vi "Mass Flow Control 8 Ch Subvi.vi"(0 "LINX In":T1, 8 "VISA resource name":refnum<visa-resource-name>="COM5", 10 "Servo Channel":u8=11, 11 "MFC 8 set point":dbl, 13 "MFC 7 set point":dbl, 14 "MFC 1  set point":dbl, 15 "MFC 2 set point":dbl, 16 "MFC 3 set point":dbl, 17 "MFC 4 set point":dbl, 18 "MFC 5 set point":dbl, 19 "MFC 6 set point":dbl) -> (12 "LINX Out":T1)   [LabVIEW 2013]
uses:
  647 Multi Gas Controller.llb/647 Open/Close Valve .vi
  <vilib>/MakerHub/LINX/Public/Sensors/Motion/Servo/Servo.lvlib
  <vilib>/Instr/_visa.llb/VISA Configure Serial Port (Instr).vi
  <vilib>/MakerHub/LINX/Public/Sensors/Motion/Servo/Servo Set Pulse Width One Channel.vi
  <vilib>/MakerHub/LINX/Private/Type Defs/Platform.ctl
  <vilib>/MakerHub/LINX/LMH-LINX.lvlib
  <vilib>/MakerHub/LINX/Private/Type Defs/Interface.ctl
  <vilib>/MakerHub/LINX/Private/Device/Type Defs/TCP Config.ctl
  <vilib>/MakerHub/LINX/Private/Device/Device.lvlib
  <vilib>/MakerHub/LINX/Private/Device/Type Defs/Channels.ctl
  <vilib>/MakerHub/LINX/Private/Device/Type Defs/LINX Device Config.ctl
  <vilib>/MakerHub/LINX/Private/Type Defs/LINX Ref.ctl
panel:
  in  "Off":dbl=1900.0
  in  "On":dbl=860.0
  out "GCF 8":dbl=1.0
  out "GCF 7":dbl=1.0
  out "GCF 6":dbl=1.0
  out "MFC 8 Size":dbl=1.0
  out "MFC 7 Size":dbl=1.0
  out "MFC 6 Size":dbl=1.0
  out "MFC 8 Status":bool
  out "MFC 7 Status":bool
  out "MFC 6 Status":bool
  out "GCF 5":dbl=0.94
  out "GCF 4":dbl=1.01
  out "GCF 3":dbl=1.22
  out "GCF 2":dbl=0.9
  out "GCF 1":dbl=0.95
  out "MFC 5 Size":dbl=100.0
  out "MFC 4 Size":dbl=50.0
  out "MFC 3 Size":dbl=50.0
  out "MFC 2 Size":dbl=100.0
  out "MFC 1 Size":dbl=50.0
  out "MFC 5 Status":bool
  out "MFC 4 Status":bool
  out "MFC 1 Status":bool
  out "MFC 2 Status":bool
  out "MFC 3 Status":bool
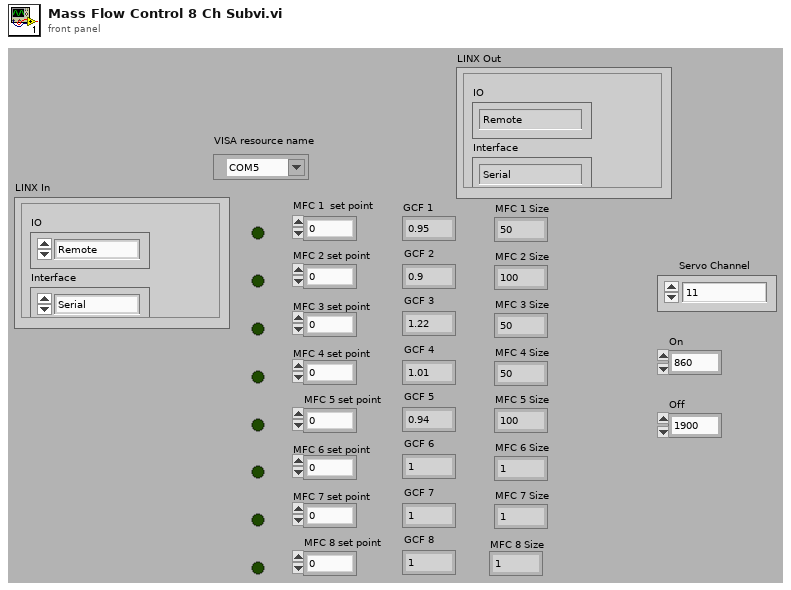
[diagram p1: front panel]
types:
  T1 = typedef "LMH-LINX.lvlib/LINX Ref.ctl" = cluster{"IO":T2, "Interface":T3, "LINX Device Config":T4}
  T2 = typedef "LMH-LINX.lvlib/Platform.ctl" = enum16{"Remote", "Local"}
  T3 = typedef "LMH-LINX.lvlib/Interface.ctl" = enum16{"Serial", "TCP"}
  T4 = typedef "LMH-LINX.lvlib/Device.lvlib/LINX Device Config.ctl" = cluster{"Interface":T3, "COM Port":refnum<visa-resource-name>, "TCP Configuration":T5, "Device Family":u8, "Device ID":u8, "Device Name":string, "TCP Ref":refnum<k5>, "Channels":T6}
  T5 = typedef "LMH-LINX.lvlib/Device.lvlib/TCP Config.ctl" = cluster{"IP Address":string, "Port":u16}
  T6 = typedef "LMH-LINX.lvlib/Channels.ctl" = cluster{"DI":u8[], "DO":u8[], "AI":u8[], "AO":u8[], "PWM":u8[], "QE":u8[], "UART":u8[], "I2C 2":u8[], "SPI":u8[], "CAN":u8[], "Servo":u8[], "AI Ref (V)":dbl, "AI Resolution (Bits)":u8, "AO Ref (V)":dbl, "AO Resolution (Bits)":u8}
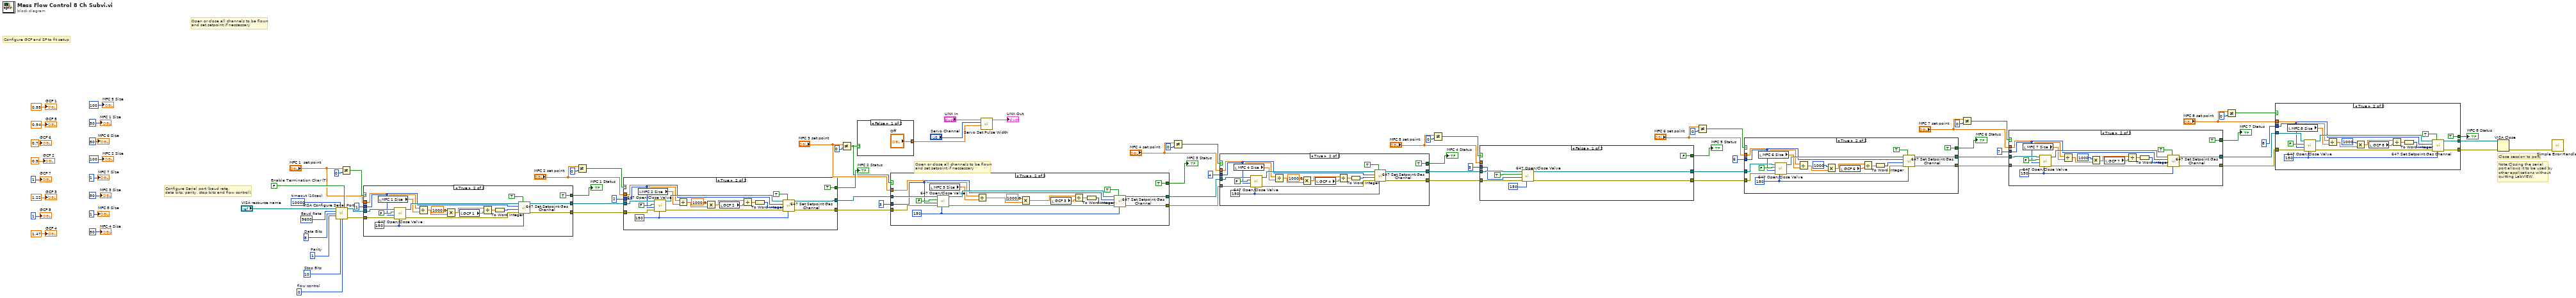
[diagram p0: block diagram]
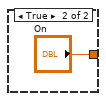
[diagram p2: hidden frame]
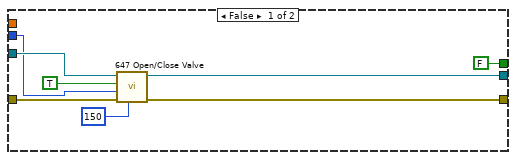
[diagram p3: hidden frame]
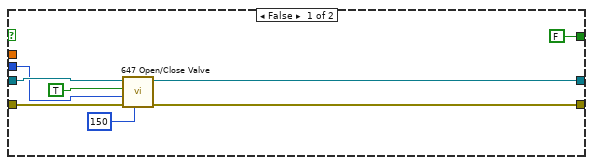
[diagram p4: hidden frame]
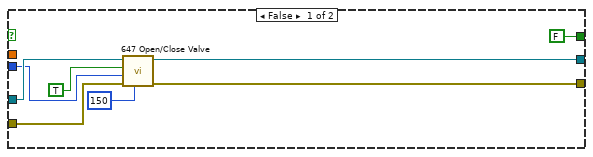
[diagram p5: hidden frame]
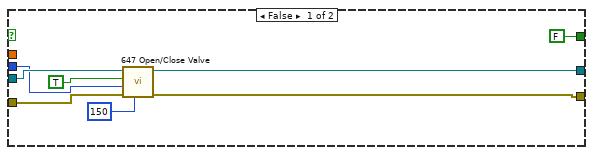
[diagram p6: hidden frame]
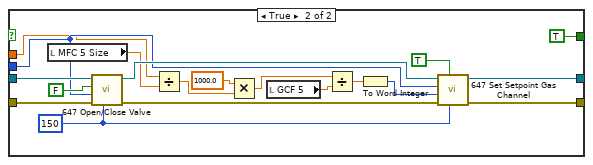
[diagram p7: hidden frame]
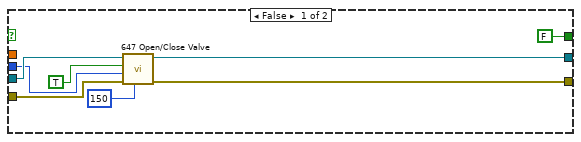
[diagram p8: hidden frame]
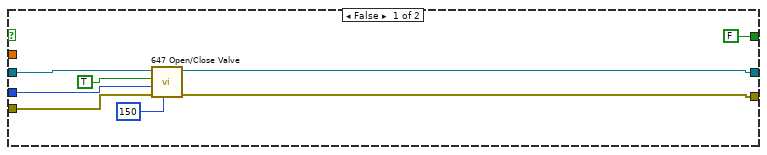
[diagram p9: hidden frame]
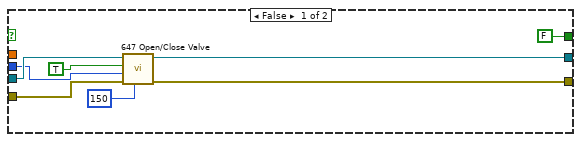
[diagram p10: hidden frame]
diagram:
  w80 = 0  # flow control
  w81 = 10  # Stop Bits
  w82 = 1  # Parity
  w83 = 8  # Data Bits
  w84 = 9600  # Baud Rate
  w85 = FALSE  # Enable Termination Char (T)
  w86 = u32 10000  # timeout (10sec)
  # "Open or close all channels to be flown\nand set setpoint if neccessary"
  # "Open or close all channels to be flown\nand set setpoint if neccessary"
  # "Configure GCF and SF to fit setup"
  # "Note:Closing the serial port allows it to be used by other applications without\nquitting LabVIEW."
  # "Close session to port."
  # "Configure Serial port (baud rate,\ndata bits, parity, stop bits and flow control)."
  n1 = call-poly "VISA Configure Serial Port"("VISA resource name"="VISA resource name", "timeout (10sec)"=w86, "Enable Termination\nChar (T)"=w85, "baud rate (9600)"=w84, "data bits (8)"=w83, "parity (0:none)"=w82, "stop bits (10: 1 bit)"=w81, "flow control (0:none)"=w80) -> ("VISA resource name out"=w79:refnum<visa-resource-name>, "error out"=w78:errorcluster)  [unwired: 6 in]
  n2 = Not Equal?(x="MFC 1  set point", y=0) -> (x != y?=w26:bool)
  n3 = case shown="True" w26 {
    tunnel: w78 -> [w91 w114]
    tunnel: [w92 w109] -> w69
    tunnel: w79 -> [w94 w113]
    tunnel: [w93 w110] -> w70
    tunnel: 1 -> [w90 w99]
    tunnel: [FALSE TRUE] -> w64
    tunnel: "MFC 1  set point" -> [_ w96]
    frame False {
      n4 = call "647 Open/Close Valve .vi"("ms Wartezeit"=u32 150, "error in (no error)"=w91, "Channel number"=w90, "OPEN / CLOSE"=TRUE, "VISA session"=w94) -> ("error out"=w92:errorcluster, "dup VISA session"=w93:refnum<visa-resource-name>)  [unwired: 4 in, 1 out]
    }
    frame True {
      w107 = 150
      n5 = local read "MFC 1 Size"() -> (w97:dbl)
      n6 = call "647 Open/Close Valve .vi"("ms Wartezeit"=w107, "error in (no error)"=w114, "Channel number"=w99, "OPEN / CLOSE"=FALSE, "VISA session"=w113) -> ("error out"=w108:errorcluster, "dup VISA session"=w111:refnum<visa-resource-name>)  [unwired: 4 in, 1 out]
      n7 = Divide(x=w96, y=w97) -> (x/y=w102:dbl)
      n8 = Multiply(x=1000.0, y=w102) -> (x*y=w100:dbl)
      n9 = local read "GCF 1"() -> (w98:dbl)
      n10 = Divide(x=w100, y=w98) -> (x/y=w101:dbl)
      n11 = To Word Integer(number=w101) -> (16bit integer=w105:i16)
      n12 = call "647 Set Setpoint Gas Channel.vi"("ms Wartezeit"=w107, "Read / Write"=TRUE, "error in (no error)"=w108, "Setpoint 0..1100\n0.1% F.S. MFC"=w105, "Channel number"=w99, "VISA session"=w111) -> ("error out"=w109:errorcluster, "dup VISA session"=w110:refnum<visa-resource-name>)  [unwired: 3 in, 1 out]
    }
  }
  "MFC 1 Status" <- w64
  n13 = Not Equal?(x="MFC 2 set point", y=0) -> (x != y?=w23:bool)
  n14 = case shown="True" w23 {
    tunnel: w70 -> [w120 w141]
    tunnel: w69 -> [w119 w140]
    tunnel: [w118 w137] -> w68
    tunnel: [w117 w136] -> w67
    tunnel: 2 -> [w116 w130]
    tunnel: [FALSE TRUE] -> w65
    tunnel: "MFC 2 set point" -> [_ w123]
    frame False {
      n15 = call "647 Open/Close Valve .vi"("ms Wartezeit"=u32 150, "error in (no error)"=w119, "Channel number"=w116, "OPEN / CLOSE"=TRUE, "VISA session"=w120) -> ("error out"=w118:errorcluster, "dup VISA session"=w117:refnum<visa-resource-name>)  [unwired: 4 in, 1 out]
    }
    frame True {
      w134 = 150
      n16 = local read "MFC 2 Size"() -> (w125:dbl)
      n17 = call "647 Open/Close Valve .vi"("ms Wartezeit"=w134, "error in (no error)"=w140, "Channel number"=w130, "OPEN / CLOSE"=FALSE, "VISA session"=w141) -> ("error out"=w138:errorcluster, "dup VISA session"=w135:refnum<visa-resource-name>)  [unwired: 4 in, 1 out]
      n18 = Divide(x=w123, y=w125) -> (x/y=w129:dbl)
      n19 = Multiply(x=1000.0, y=w129) -> (x*y=w126:dbl)
      n20 = local read "GCF 2"() -> (w124:dbl)
      n21 = Divide(x=w126, y=w124) -> (x/y=w127:dbl)
      n22 = To Word Integer(number=w127) -> (16bit integer=w132:i16)
      n23 = call "647 Set Setpoint Gas Channel.vi"("ms Wartezeit"=w134, "Read / Write"=TRUE, "error in (no error)"=w138, "Setpoint 0..1100\n0.1% F.S. MFC"=w132, "Channel number"=w130, "VISA session"=w135) -> ("error out"=w137:errorcluster, "dup VISA session"=w136:refnum<visa-resource-name>)  [unwired: 3 in, 1 out]
    }
  }
  "MFC 2 Status" <- w65
  n24 = Not Equal?(x="MFC 3 set point", y=0) -> (x != y?=w13:bool)
  n25 = case shown="False" w13 {
    tunnel: ["Off" "On"] -> w28
    frame False {
    }
    frame True {
    }
  }
  n26 = case shown="True" w13 {
    tunnel: w68 -> [w149 w170]
    tunnel: [w150 w164] -> w74
    tunnel: w67 -> [w148 w169]
    tunnel: [w151 w167] -> w72
    tunnel: 3 -> [w146 w158]
    tunnel: [FALSE TRUE] -> w66
    tunnel: "MFC 3 set point" -> [_ w152]
    frame False {
      n27 = call "647 Open/Close Valve .vi"("ms Wartezeit"=u32 150, "error in (no error)"=w149, "Channel number"=w146, "OPEN / CLOSE"=TRUE, "VISA session"=w148) -> ("error out"=w150:errorcluster, "dup VISA session"=w151:refnum<visa-resource-name>)  [unwired: 4 in, 1 out]
    }
    frame True {
      w163 = 150
      n28 = local read "MFC 3 Size"() -> (w154:dbl)
      n29 = call "647 Open/Close Valve .vi"("ms Wartezeit"=w163, "error in (no error)"=w170, "Channel number"=w158, "OPEN / CLOSE"=FALSE, "VISA session"=w169) -> ("error out"=w165:errorcluster, "dup VISA session"=w166:refnum<visa-resource-name>)  [unwired: 4 in, 1 out]
      n30 = Divide(x=w152, y=w154) -> (x/y=w161:dbl)
      n31 = Multiply(x=1000.0, y=w161) -> (x*y=w155:dbl)
      n32 = local read "GCF 3"() -> (w153:dbl)
      n33 = Divide(x=w155, y=w153) -> (x/y=w156:dbl)
      n34 = To Word Integer(number=w156) -> (16bit integer=w160:i16)
      n35 = call "647 Set Setpoint Gas Channel.vi"("ms Wartezeit"=w163, "Read / Write"=TRUE, "error in (no error)"=w165, "Setpoint 0..1100\n0.1% F.S. MFC"=w160, "Channel number"=w158, "VISA session"=w166) -> ("error out"=w164:errorcluster, "dup VISA session"=w167:refnum<visa-resource-name>)  [unwired: 3 in, 1 out]
    }
  }
  "MFC 3 Status" <- w66
  n36 = call-poly <vilib>:"Servo Set Pulse Width.vi"("Pulse Width (uS)"=w28, "Servo Channel"="Servo Channel", "LINX Resource"="LINX In") -> ("LINX Resource"=→"LINX Out":T1)  [unwired: 7 in, 1 out]
  n37 = Not Equal?(x="MFC 4 set point", y=0) -> (x != y?=w18:bool)
  n38 = case shown="True" w18 {
    tunnel: w74 -> [w178 w196]
    tunnel: [w177 w192] -> w73
    tunnel: w72 -> [w176 w197]
    tunnel: [w175 w193] -> w71
    tunnel: [FALSE TRUE] -> w63
    tunnel: 4 -> [w171 w184]
    tunnel: "MFC 4 set point" -> [_ w179]
    frame False {
      n39 = call "647 Open/Close Valve .vi"("ms Wartezeit"=u32 150, "error in (no error)"=w178, "Channel number"=w171, "OPEN / CLOSE"=TRUE, "VISA session"=w176) -> ("error out"=w177:errorcluster, "dup VISA session"=w175:refnum<visa-resource-name>)  [unwired: 4 in, 1 out]
    }
    frame True {
      w190 = u32 150
      n40 = local read "MFC 4 Size"() -> (w182:dbl)
      n41 = call "647 Open/Close Valve .vi"("ms Wartezeit"=w190, "error in (no error)"=w196, "Channel number"=w184, "OPEN / CLOSE"=FALSE, "VISA session"=w197) -> ("error out"=w191:errorcluster, "dup VISA session"=w194:refnum<visa-resource-name>)  [unwired: 4 in, 1 out]
      n42 = Divide(x=w179, y=w182) -> (x/y=w188:dbl)
      n43 = Multiply(x=1000.0, y=w188) -> (x*y=w180:dbl)
      n44 = local read "GCF 4"() -> (w181:dbl)
      n45 = Divide(x=w180, y=w181) -> (x/y=w183:dbl)
      n46 = To Word Integer(number=w183) -> (16bit integer=w187:i16)
      n47 = call "647 Set Setpoint Gas Channel.vi"("ms Wartezeit"=w190, "Read / Write"=TRUE, "error in (no error)"=w191, "Setpoint 0..1100\n0.1% F.S. MFC"=w187, "Channel number"=w184, "VISA session"=w194) -> ("error out"=w192:errorcluster, "dup VISA session"=w193:refnum<visa-resource-name>)  [unwired: 3 in, 1 out]
    }
  }
  "MFC 4 Status" <- w63
  n48 = Not Equal?(x="MFC 5 set point", y=0) -> (x != y?=w14:bool)
  n49 = case shown="False" w14 {
    tunnel: w73 -> [w205 w223]
    tunnel: w71 -> [w204 w224]
    tunnel: [FALSE TRUE] -> w62
    tunnel: 5 -> [w200 w213]
    tunnel: [w198 w210] -> w46
    tunnel: [w199 w209] -> w45
    tunnel: "MFC 5 set point" -> [_ w206]
    frame False {
      n50 = call "647 Open/Close Valve .vi"("ms Wartezeit"=u32 150, "error in (no error)"=w205, "Channel number"=w200, "OPEN / CLOSE"=TRUE, "VISA session"=w204) -> ("error out"=w199:errorcluster, "dup VISA session"=w198:refnum<visa-resource-name>)  [unwired: 4 in, 1 out]
    }
    frame True {
      w219 = u32 150
      n51 = local read "MFC 5 Size"() -> (w208:dbl)
      n52 = call "647 Open/Close Valve .vi"("ms Wartezeit"=w219, "error in (no error)"=w223, "Channel number"=w213, "OPEN / CLOSE"=FALSE, "VISA session"=w224) -> ("error out"=w220:errorcluster, "dup VISA session"=w221:refnum<visa-resource-name>)  [unwired: 4 in, 1 out]
      n53 = Divide(x=w206, y=w208) -> (x/y=w217:dbl)
      n54 = Multiply(x=1000.0, y=w217) -> (x*y=w212:dbl)
      n55 = local read "GCF 5"() -> (w207:dbl)
      n56 = Divide(x=w212, y=w207) -> (x/y=w211:dbl)
      n57 = To Word Integer(number=w211) -> (16bit integer=w216:i16)
      n58 = call "647 Set Setpoint Gas Channel.vi"("ms Wartezeit"=w219, "Read / Write"=TRUE, "error in (no error)"=w220, "Setpoint 0..1100\n0.1% F.S. MFC"=w216, "Channel number"=w213, "VISA session"=w221) -> ("error out"=w209:errorcluster, "dup VISA session"=w210:refnum<visa-resource-name>)  [unwired: 3 in, 1 out]
    }
  }
  "MFC 5 Status" <- w62
  n59 = Not Equal?(x="MFC 6 set point", y=0) -> (x != y?=w10:bool)
  n60 = case shown="True" w10 {
    tunnel: [FALSE TRUE] -> w56
    tunnel: [w231 w246] -> w53
    tunnel: [w229 w245] -> w51
    tunnel: 6 -> [w227 w244]
    tunnel: w46 -> [w230 w242]
    tunnel: w45 -> [w232 w241]
    tunnel: "MFC 6 set point" -> [_ w233]
    frame False {
      n61 = call "647 Open/Close Valve .vi"("ms Wartezeit"=150, "error in (no error)"=w232, "Channel number"=w227, "OPEN / CLOSE"=TRUE, "VISA session"=w230) -> ("error out"=w231:errorcluster, "dup VISA session"=w229:refnum<visa-resource-name>)  [unwired: 4 in, 1 out]
    }
    frame True {
      w243 = 150
      n62 = local read "MFC 6 Size"() -> (w236:dbl)
      n63 = call "647 Open/Close Valve .vi"("ms Wartezeit"=w243, "error in (no error)"=w241, "Channel number"=w244, "OPEN / CLOSE"=FALSE, "VISA session"=w242) -> ("error out"=w249:errorcluster, "dup VISA session"=w248:refnum<visa-resource-name>)  [unwired: 4 in, 1 out]
      n64 = Divide(x=w233, y=w236) -> (x/y=w240:dbl)
      n65 = Multiply(x=1000, y=w240) -> (x*y=w234:dbl)
      n66 = local read "GCF 6"() -> (w235:dbl)
      n67 = Divide(x=w234, y=w235) -> (x/y=w238:dbl)
      n68 = To Word Integer(number=w238) -> (16bit integer=w237:i16)
      n69 = call "647 Set Setpoint Gas Channel.vi"("ms Wartezeit"=w243, "Read / Write"=TRUE, "error in (no error)"=w249, "Setpoint 0..1100\n0.1% F.S. MFC"=w237, "Channel number"=w244, "VISA session"=w248) -> ("error out"=w246:errorcluster, "dup VISA session"=w245:refnum<visa-resource-name>)  [unwired: 3 in, 1 out]
    }
  }
  "MFC 6 Status" <- w56
  n70 = Not Equal?(x="MFC 7 set point", y=0) -> (x != y?=w6:bool)
  n71 = case shown="True" w6 {
    tunnel: [FALSE TRUE] -> w55
    tunnel: w53 -> [w259 w273]
    tunnel: [w258 w272] -> w52
    tunnel: w51 -> [w257 w271]
    tunnel: [w256 w270] -> w50
    tunnel: 7 -> [w254 w269]
    tunnel: "MFC 7 set point" -> [_ w260]
    frame False {
      n72 = call "647 Open/Close Valve .vi"("ms Wartezeit"=150, "error in (no error)"=w259, "Channel number"=w254, "OPEN / CLOSE"=TRUE, "VISA session"=w257) -> ("error out"=w258:errorcluster, "dup VISA session"=w256:refnum<visa-resource-name>)  [unwired: 4 in, 1 out]
    }
    frame True {
      w268 = 150
      n73 = local read "MFC 7 Size"() -> (w263:dbl)
      n74 = call "647 Open/Close Valve .vi"("ms Wartezeit"=w268, "error in (no error)"=w273, "Channel number"=w269, "OPEN / CLOSE"=FALSE, "VISA session"=w271) -> ("error out"=w276:errorcluster, "dup VISA session"=w277:refnum<visa-resource-name>)  [unwired: 4 in, 1 out]
      n75 = Divide(x=w260, y=w263) -> (x/y=w267:dbl)
      n76 = Multiply(x=1000, y=w267) -> (x*y=w262:dbl)
      n77 = local read "GCF 7"() -> (w261:dbl)
      n78 = Divide(x=w262, y=w261) -> (x/y=w265:dbl)
      n79 = To Word Integer(number=w265) -> (16bit integer=w264:i16)
      n80 = call "647 Set Setpoint Gas Channel.vi"("ms Wartezeit"=w268, "Read / Write"=TRUE, "error in (no error)"=w276, "Setpoint 0..1100\n0.1% F.S. MFC"=w264, "Channel number"=w269, "VISA session"=w277) -> ("error out"=w272:errorcluster, "dup VISA session"=w270:refnum<visa-resource-name>)  [unwired: 3 in, 1 out]
    }
  }
  "MFC 7 Status" <- w55
  n81 = Not Equal?(x="MFC 8 set point", y=0) -> (x != y?=w4:bool)
  n82 = case shown="True" w4 {
    tunnel: [FALSE TRUE] -> w54
    tunnel: w52 -> [w286 w300]
    tunnel: w50 -> [w284 w299]
    tunnel: 8 -> [w281 w298]
    tunnel: [w285 w296] -> w76
    tunnel: [w283 w291] -> w75
    tunnel: "MFC 8 set point" -> [_ w287]
    frame False {
      n83 = call "647 Open/Close Valve .vi"("ms Wartezeit"=150, "error in (no error)"=w286, "Channel number"=w281, "OPEN / CLOSE"=TRUE, "VISA session"=w284) -> ("error out"=w285:errorcluster, "dup VISA session"=w283:refnum<visa-resource-name>)  [unwired: 4 in, 1 out]
    }
    frame True {
      w297 = 150
      n84 = local read "MFC 8 Size"() -> (w290:dbl)
      n85 = call "647 Open/Close Valve .vi"("ms Wartezeit"=w297, "error in (no error)"=w300, "Channel number"=w298, "OPEN / CLOSE"=FALSE, "VISA session"=w299) -> ("error out"=w303:errorcluster, "dup VISA session"=w304:refnum<visa-resource-name>)  [unwired: 4 in, 1 out]
      n86 = Divide(x=w287, y=w290) -> (x/y=w295:dbl)
      n87 = Multiply(x=1000, y=w295) -> (x*y=w288:dbl)
      n88 = local read "GCF 8"() -> (w289:dbl)
      n89 = Divide(x=w288, y=w289) -> (x/y=w293:dbl)
      n90 = To Word Integer(number=w293) -> (16bit integer=w292:i16)
      n91 = call "647 Set Setpoint Gas Channel.vi"("ms Wartezeit"=w297, "Read / Write"=TRUE, "error in (no error)"=w303, "Setpoint 0..1100\n0.1% F.S. MFC"=w292, "Channel number"=w298, "VISA session"=w304) -> ("error out"=w296:errorcluster, "dup VISA session"=w291:refnum<visa-resource-name>)  [unwired: 3 in, 1 out]
    }
  }
  "MFC 8 Status" <- w54
  n92 = VISA Close(VISA resource name=w75, error in (no error)=w76) -> (error out=w77:errorcluster)
  n93 = call <vilib>:"Simple Error Handler.vi"("error in (no error)"=w77) -> ()  [unwired: 4 in, 5 out]
  "MFC 1 Size" <- 50
  "GCF 1" <- 0.95
  "MFC 2 Size" <- 100
  "GCF 2" <- 0.9
  "MFC 3 Size" <- 50
  "GCF 3" <- 1.22
  "MFC 4 Size" <- 50
  "GCF 4" <- 1.47
  "MFC 5 Size" <- 100
  "GCF 5" <- 0.94
  "GCF 6" <- 0.7
  "MFC 6 Size" <- 50
  "MFC 7 Size" <- 1
  "MFC 8 Size" <- 1
  "GCF 7" <- 1
  "GCF 8" <- 1
